vi "class_data.vi"() -> ()   [LabVIEW 2010, in "ErrorController.lvclass"]
uses:
  ErrorController.lvclass
  queue controller.ctl
  error_cluster.ctl
panel:
  out "error queue":T1
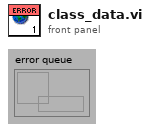
[diagram p1: front panel]
types:
  T1 = typedef "ErrorController.lvclass/queue controller.ctl" = refnum<queue>
diagram:
